vi "execute_value_write_policy.vi"(8 "error in (no error)":errorcluster, 9 "Publish Time":timestamp, 10 "New Topic Value":variant, 11 "ValueChangeSubscription In":refnum<class "ValueChangeSubscription.lvclass">) -> (0 "error out":errorcluster, 3 "ValueChangeSubscription Out":refnum<class "ValueChangeSubscription.lvclass">)   [LabVIEW 2015, in "SubscriptionPolicy.lvlib" / "ValueChangeSubscription.lvclass"]
uses:
  ValueChangeSubscription.lvclass
  ValueChangeSubscription.lvclass/ValueChangeSubscription.ctl
  IMediator/ISubscriptionPolicy/ISubscriptionPolicy.lvclass/ISubscriptionPolicy.ctl
  IMediator/ITransport/ITransport.lvclass
  IMediator/ISubscriptionPolicy/ISubscriptionPolicy.lvclass
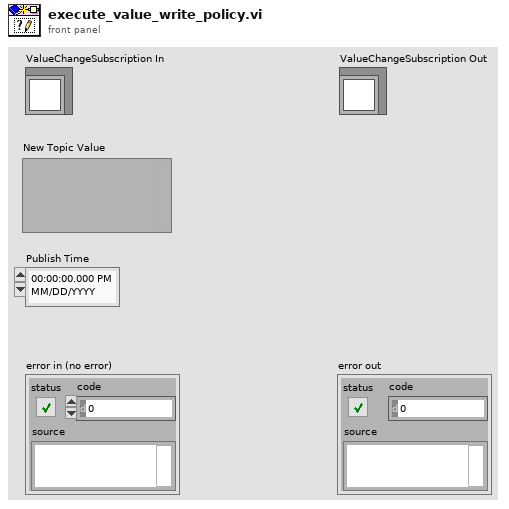
[diagram p1: front panel]
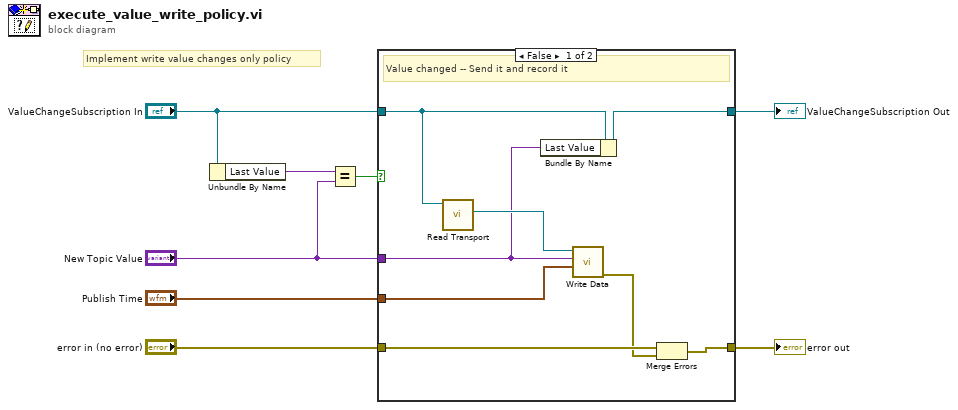
[diagram p0: block diagram]
diagram:
  # "Implement write value changes only policy"
  n1 = Unbundle By Name("ValueChangeSubscription In") -> ("Last Value"=w4:variant)
  n2 = Equal?(x=w4, y="New Topic Value") -> (x = y?=w3:bool)
  n3 = case shown="False" w3 {
    tunnel: "New Topic Value" -> [w9 _]
    tunnel: "Publish Time" -> [w16 _]
    tunnel: "error in (no error)" -> [w15 w17]
    tunnel: [w14 w17] -> w5
    tunnel: "ValueChangeSubscription In" -> [w12 w18]
    tunnel: [w10 w18] -> w1
    frame False {
      # "Value changed -- Send it and record it"
      n4 = call "Read Transport.vi"("ISubscriptionPolicy in"=w12) -> ("Transport"=w11:refnum<class "ITransport.lvclass">)  [unwired: 10 in]
      n5 = Bundle By Name(cluster=w12, "Last Value"=w9) -> (w10:refnum<class "ValueChangeSubscription.lvclass">)
      n6 = call-dynamic "Write Data.vi"("Publication Time"=w16, "Value"=w9, "ITransport in"=w11) -> ("error out"=w13:errorcluster)  [unwired: 7 in, 1 out]
      n7 = Merge Errors(w15, w13) -> (w14:errorcluster)
    }
    frame True {
      # "No value change -- Do nothing"
    }
  }
  "error out" <- w5
  "ValueChangeSubscription Out" <- w1
